vi "Union Unified Msg Set.vi"(11 "Get Actor in":refnum<class "Actor.lvclass">) -> (2 "Unified Msg Set":T1)   [LabVIEW 2025, in "jettl.lvlib" / "Actor.lvlib" / "Actor.lvclass"]
uses:
  Actor.lvclass
  Msg Set.ctl
  Msg/Msg.lvclass
  Actor.lvlib
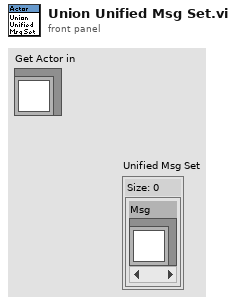
[diagram p1: front panel]
types:
  T1 = typedef "jettl.lvlib/Actor.lvlib/Msg Set.ctl" = set{refnum<class "Msg.lvclass">}
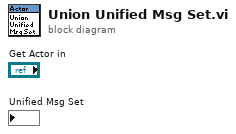
[diagram p0: block diagram]
diagram:
